vi "Save_Info.vi"(8 "error in (no error)":errorcluster, 11 "AB_DLL in":refnum<class "AB_DLL.lvclass">) -> (0 "error out":errorcluster, 3 "AB_DLL out":refnum<class "AB_DLL.lvclass">)   [LabVIEW 2020, in "AB_DLL.lvclass"]
uses:
  <vilib>/AppBuilder/AB_Classes/DLL/AB_DLL.lvclass
  e:/builds/penguin/labview/branches/2020/dev/dist/vi.lib/AppBuilder/AB_Classes/Build/AB_Build.lvclass
  <vilib>/AppBuilder/RW_Project/AB_RW_Project_PropBag_Action.ctl
  <vilib>/AppBuilder/AB_Classes/DLL/AB_DLL.lvclass/AB_DLL.ctl
  <vilib>/AppBuilder/AB_Classes/Application/AB_Application.lvclass
  <vilib>/AppBuilder/AB_Classes/Build/AB_Build.lvclass
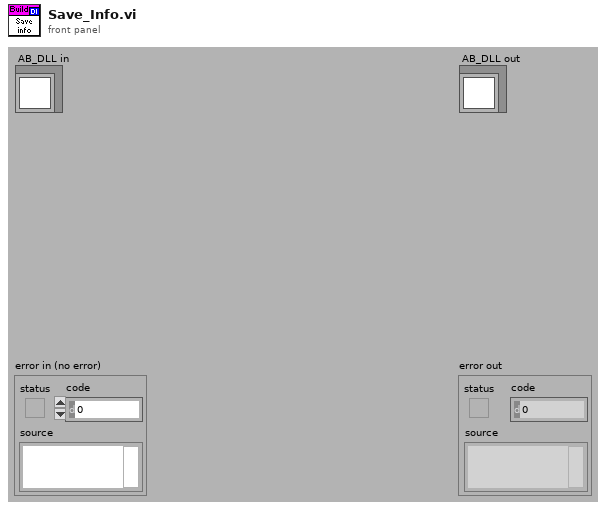
[diagram p1: front panel]
types:
  T1 = typedef "AB_RW_Project_PropBag_Action.ctl" = enum16{"read", "write", "clear", "readPrevious", "writePrevious", "clearPrevious"}
  T2 = typedef "AB_DLL.ctl" = cluster{"delayOSMsg":bool, "includeHeaders":bool, "embeddedRTE":bool, "headerGUID":string, "libGUID":string, "compatibilityWith2011":bool, "includeTypeLibrary":bool, "privateExecutionSystem":bool}
  T3 = typedef "AB_Build.ctl" = cluster{"buildSpecName":string, "buildSpecDescription":string, "destinations":refnum<class "AB_Destination.lvclass">[], "exclusionOption":T4, "defaultLanguage":string, "supportedLanguages":string[], "excludedDirectories":path[], "buildContext":refnum<vi>, "buildObject":T5, "preview":bool, "programatic":bool, "progressBarEvents":T6, "userLog_Path":path, "preActionID":string, "preAction_Path":path, "postActionID":string, "postAction_Path":path, "eng_checkForBrokenVIs?":bool, "eng_verboseLinkerErrors?":bool, "localDest_Path":path, "targetDest_Path":path, "removeVIObject":u16, "cache":refnum<class "PreviewCache.lvclass">, "use cache":bool, "previewCache_ID":string, "buildCache_ID":string, "eng_TempLocalDest_Path":path, "eng_collectDependencies?":bool, "versionInfo":cluster{"buildVersion":cluster{"major":u16, "minor":u16, "patch":u16, "build":u16}, "autoIncrement":bool}, "eng_enableVIChecksums":bool}
  T4 = typedef "AB_Exclusion_Option.ctl" = cluster{"typedefs":bool, "polymorphicVIs":bool, "unusedLibraryItems":bool, "modifyLibraryFile":bool, "edit-timeDependencies":bool, "inlineVIs":bool, "dependent PPLs":bool, "dependent DLLs":bool}
  T5 = typedef "ItemRef.ctl" = u64
  T6 = typedef "provcom_ProgressBar_Events.ctl" = cluster{"newJob":refnum<user-event>, "newItem":refnum<user-event>, "errorMsg":T7, "cancel":refnum<user-event>}
  T7 = typedef "mxLvBuildError.ctl" = refnum<user-event>
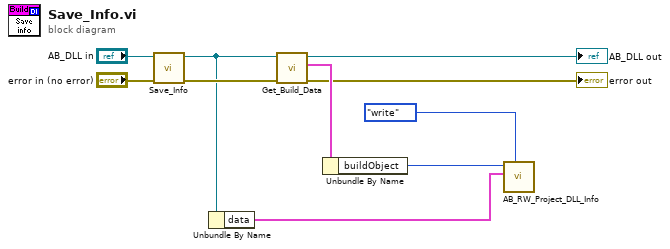
[diagram p0: block diagram]
diagram:
  n1 = call-parent "Save_Info.vi"("error in (no error)"="error in (no error)", "AB_Application in"="AB_DLL in") -> ("error out"=w6:errorcluster, "AB_Application out"=w4:refnum<class "AB_DLL.lvclass">)  [unwired: 8 in]
  n2 = Unbundle By Name(w4) -> ("data"=w2:T2)
  n3 = call <vilib>:"Get_Build_Data.vi"("error in (no error)"=w6, "Class in"=w4) -> ("error out"=→"error out":errorcluster, "data"=w8:T3, "Class out"=→"AB_DLL out":refnum<class "AB_DLL.lvclass">)  [unwired: 7 in]
  n4 = Unbundle By Name(w8) -> ("buildObject"=w1:T5)
  n5 = call <vilib>:"AB_RW_Project_DLL_Info.vi"("action"=AB_RW_Project_PropBag_Action."write", "Dll_info in"=w2, "Object In"=w1) -> ()  [unwired: 6 in, 3 out]
